vi "Forebrain.vi"() -> ()   [LabVIEW 2010]
doc: "This VI contrains the Forebrain within the Olin Robot Architecture. It must be run first to load the appropriate mission definition files. It contains a finite state machine built around a tabbed Operator interface that will guide an operator through the startup, run shutdown mission sequence. After running it, run the Midbrain and Hindbrain VIS."
panel:
  out "MDF_Original":T1(array[cluster])
  out "(xr,yr) A":cluster{"X":dbl, "Y":dbl}
  out "What?Midbrain":cluster{"T":dbl, "Range":dbl, "Bearing":dbl}[](array[cluster])
  out "How?Midbrain":cluster{"T":dbl, "Battery":dbl, "Temp":dbl}
  out "What?Forebrain":cluster{"T":dbl, "Range":dbl, "Bearing":dbl}[](array[cluster])
  out "How?Forebrain":cluster{"T":dbl, "Battery":dbl, "Temp":dbl}
  out "Where? Forebrain":T2
  out "WhereAmI? Clean":T2
  out "(xr,yr)":cluster{"X":dbl, "Y":dbl}
  out "How?ForebrainOut":cluster{"T":dbl, "Battery":dbl, "Temp":dbl}
  out "How?MidbrainMM":cluster{"T":dbl, "Battery":dbl, "Temp":dbl}
  out "WhereAmI?MidB":T2
  out "Where?Forebrain":T2
  out "WhatAroundMe?MidB":cluster{"T":dbl, "Range":dbl, "Bearing":dbl}[](array[cluster])
  in  "RunRobot":bool
  out "Robot Live":bool
  in  "E-Stop":bool
  in  "Tab":T3(tab)
  out "Boolean 3":bool
  in  "Test Tail":bool
  out "StartMissionMap":picture
  out "Boolean 2":bool
  out "Boolean":bool
  in  "Test Starboard Motor":bool
  in  "Test Port Motor":bool
  out "Motors Hot":bool
  out "BatteryState":dbl(slide) scale=16.0..24.0
  out "LIDARCheck":picture
  out "MissionTime S&S":dbl(knob) scale=0.0..10.0
  out "CollisionWarning":bool
  out "DebugLIDAR":picture
  in  "SubPosition":T4 {"xrobot" min=0.0 max=300.0; "yrobot" min=0.0 max=300.0; "heading" min=-7.0 max=7.0 step=0.01}
  in  "LIDARControl":T5
  out "LIDAR Data (r:pixel b:degrees)":cluster{"Range":dbl, "Bearing":dbl}[](array[cluster])
  in  "Stop DebugSENSE":bool
  out "MissionMap":picture
  out "MDF Out":T1(array[cluster])
  out "initialized MDF":T1(array[cluster])
  in  "MDFile":T6
  out "Way Point Index":i32
  out "InitialWaypoint":cluster{"X":i16, "Y":i16}
  in  "Pen Color":u32(colorbox)=15671808
  in  "Select Pen Attributes":T7={"Width"=1, "Style"=enum."Solid"}
  out "Draw??":bool
  out "ManualActCommand":dbl[](array[numeric])
  out "Hypo Out":cluster{"Motor1":i16, "Motor 2":i16}
  out "NeoActCom":dbl[](array[numeric])
  out "SteerAngle":dbl
  in  "Depth_Leg":dbl(slide) min=0.0 max=20.0 step=0.01
  out "MDF":T1(array[cluster])
  in  "Select Your Behavior":T8(ring)
  out "No. of Waypoints":i32
  in  "Exit Planning":bool
  out "MissionDefFile":picture
  in  "RobotSpeed_Leg":dbl(slide) min=0.0 max=4.0 step=0.01 scale=0.0..4.0
  out "BuildMDF":bool
  out "ActManual":bool
  in  "Steering":dbl(knob) min=-25.0 max=25.0 step=1.0 scale=15.0..-15.0
  out "MWhat?":bool
  out "Where? 2":bool
  out "How? 2":bool
  in  "ManualModeStop":bool
  out "ManualModeLIDAR":picture
  out "ManualMissionMap":picture
  out "CollisionLight":bool
  out "Temp Light":bool
  in  "LIDAR":bool
  in  "MAP":bool
  out "Battery":dbl(slide) scale=16.0..24.0
  in  "RobotSpeed":dbl(slide) scale=0.0..4.0
  out "MissionTime":dbl(knob) scale=0.0..10.0
  out "Roll":dbl(knob) scale=-90.0..90.0
  out "Pitch":dbl(slide) scale=-20.0..20.0
  out "Heading":cluster{dbl, dbl}(knob)={0.0, 34.390870865624734} scale=180.0..-180.0
  out "Speed":dbl(knob) scale=0.0..4.0
  in  "Reset":bool
  out "Ready":bool
  in  "Pause":bool
  in  "Rerun MDF":bool
  out "ATempLight":bool
  out "CollisionLight 2":bool
  out "Act":bool
  out "Hypo":bool
  out "Neo-C":bool
  out "How?":bool
  out "What?":bool
  out "A Pitch":dbl(slide) scale=-20.0..20.0
  out "A Roll":dbl(knob) scale=-90.0..90.0
  out "A Heading":cluster{dbl, dbl}(knob)={0.0, 34.390870865624734} scale=180.0..-180.0
  out "A Speed":dbl(knob) scale=0.0..4.0
  out "AutoBattery":dbl(slide) scale=16.0..24.0
  out "AutoModeLIDAR":picture
  out "AutoMissionMap":picture
  in  "RunAutoMode":bool
  out "MissionTimeAuto":dbl(knob) scale=0.0..10.0
  out "Where?":bool
  # "To run\nrobot,\nclick\narrow\nabove\n\nTo shut \noff \nrobot,\nclick \nbutton\nbelow."
  # "Operation Directions\n\n1)Click on Startup&\nShutdown tab.\n2) Click on Run \nArrow on menubar.\nRun Forebrain,\nMidbrain and Hindbrain.\n3) Select a mssion \nmap file when asked.\n4) Check robot is \nfully operational on\nStartup tab.\n5) Debug with debug\ntabs as required.\n6) Select ManualMode\ntab and test drive \nrobot.\n7) Select PlanMission\ntab and set up \nmission.\n8) Go to AutoMode\ntab and run mission."
  # "Turns off drive\nmotors"
  # "To operate:\n1) Run Forebrain.vi\n2) Run Midbrain.vi\n3) Run Hindbrain.vi"
  # "Use this tab\nto explore\nLIDAR\ndata and \noperation"
  # "Set \nX=130\nY=100\nto put\nrobot\nin center of\nMission\nMap"
  # "Set\nNumberOfBeams\nSensorRange\nNoise\nto\nview\nsimulated\nsensor\ndata"
  # "Directions:\n1) Select Robot Behavior for each mission leg.\n2) Select Robot Speed for leg.\n3) Select Robot Depth for leg.\n4) Click on robots current location for first waypoint.\n5) Hold down button and drag to next\nwaypoint. Click on next leg waypoint.\n6) Hold mouse button down and drag to \nnext waypoint. \n7) Click on next waypoint. Repeat for full mission.\n8) MDF will store up to 20 waypoints."
  # "MDF"
  # "Camera"
  # "AMM"
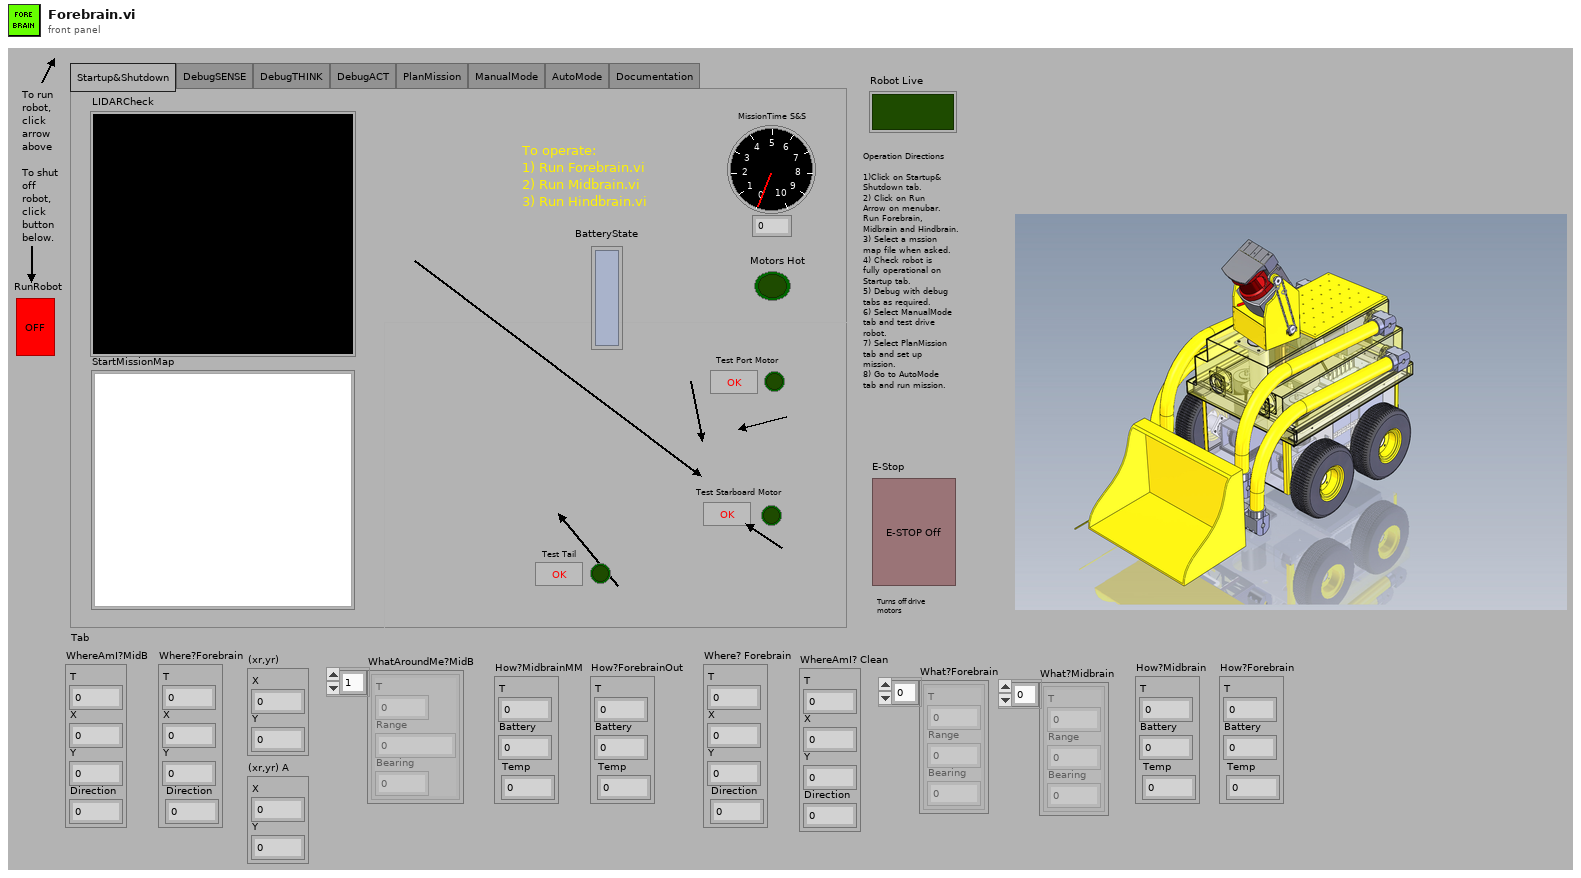
[diagram p1: front panel]
types:
  T1 = cluster{"Status":enum16{"Past", "Current", "Future"}, "x":dbl, "y":dbl, "z":dbl, "Vel":dbl, "Dwell Time":dbl, "Behavior":enum16{"OpenFieldTransit", "WallFollow", "LaneFollow", "ManualMode"}, "Expand1":dbl, "Expand2":dbl, "Expand3":dbl}[]
  T2 = cluster{"T":dbl, "X":dbl, "Y":dbl, "Direction":dbl}
  T3 = enum32{"Startup&Shutdown", "DebugSENSE", "DebugTHINK", "DebugACT", "PlanMission", "ManualMode", "AutoMode", "Documentation"}
  T4 = cluster{"xrobot":dbl, "yrobot":dbl, "heading":dbl}
  T5 = cluster{"NumberOfBeams":i32, "SensorRange":dbl, "Noise (0.1 to 1)":dbl}
  T6 = cluster{"Status":enum16{"Past", "Current", "Future"}, "x":dbl, "y":dbl, "z":dbl, "Vel":dbl, "Dwell Time":dbl, "Behavior":enum16{"OpenFieldTransit", "WallFollow", "LaneFollow", "ManualMode"}, "Expand1":dbl, "Expand2":dbl, "Expand3":dbl}
  T7 = cluster{"Width":u16, "Style":enum32{"Solid", "Dash", "Dot", "DashDot", "DashDotDot"}}
  T8 = enum16{"OpenFieldTransit", "WallFollow", "LaneFollow", "ManualMode"}
  T9 = cluster{"VelCom":dbl, "BehCom":enum16{"OpenFieldTransit", "WallFollow", "LaneFollow", "ManualMode"}}
  T10 = typedef "IMAQ Image.ctl" = refnum<image>
  T11 = typedef "imagedata.ctl" = cluster{"image type":i32, "image depth":i32, "image":u8[], "mask":u8[], "colors":u32[], "Rectangle":cluster{"left":i16, "top":i16, "right":i16, "bottom":i16}}
  T12 = typedef "LVMouseTypeDef.ctl" = cluster{"Mouse Position":cluster{"X":i32, "Y":i32}, "Mouse Modifiers":cluster{"Button Down":bool, "Shift Mod":bool, "Menu Mod":bool, "Option Mod":bool}}
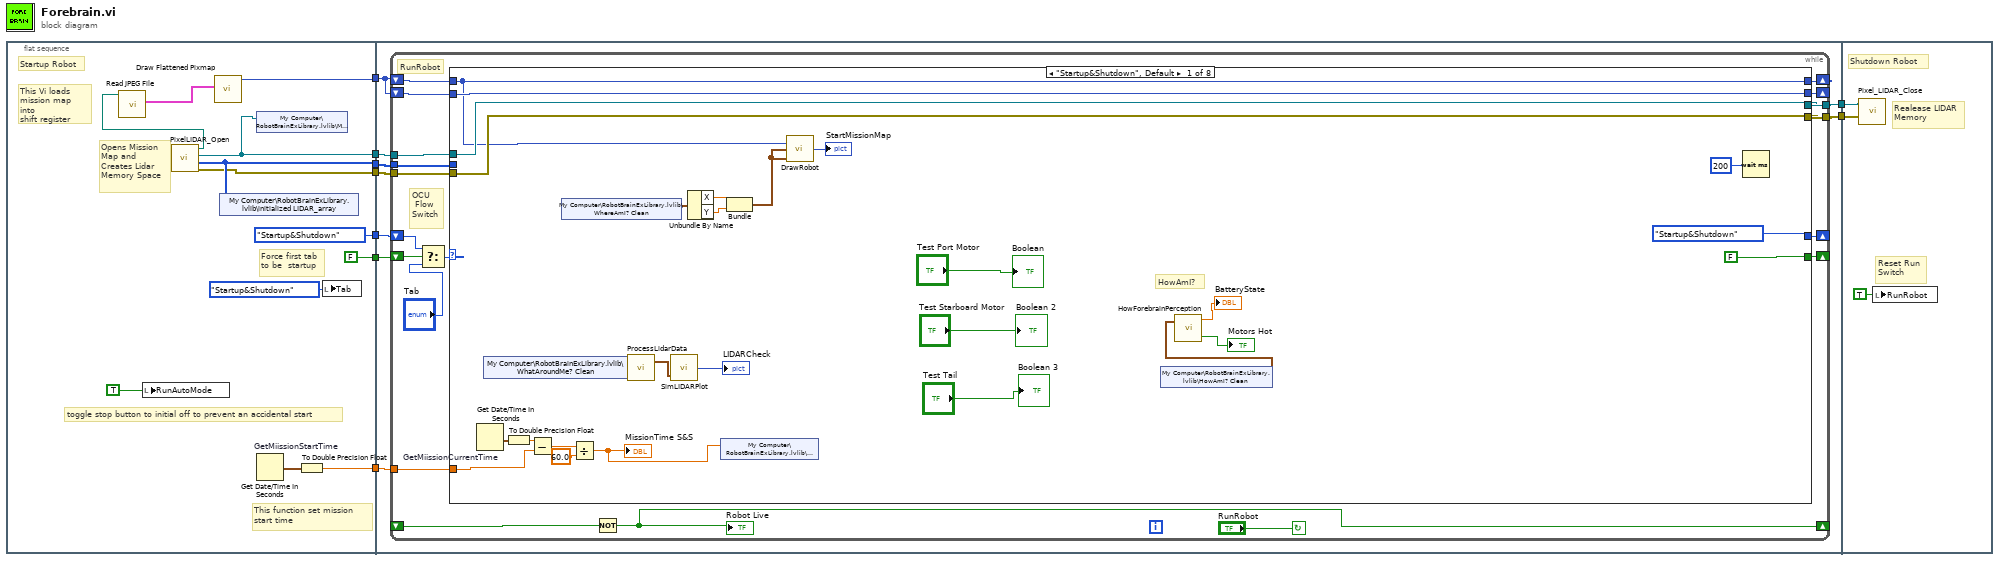
[diagram p0: block diagram]
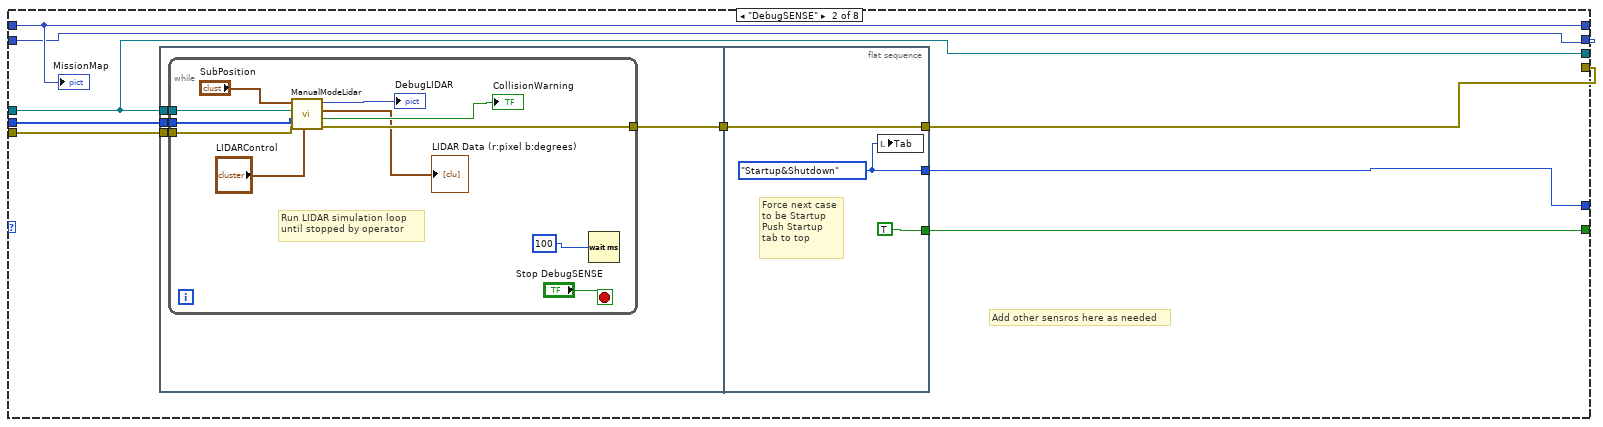
[diagram p2: hidden frame]
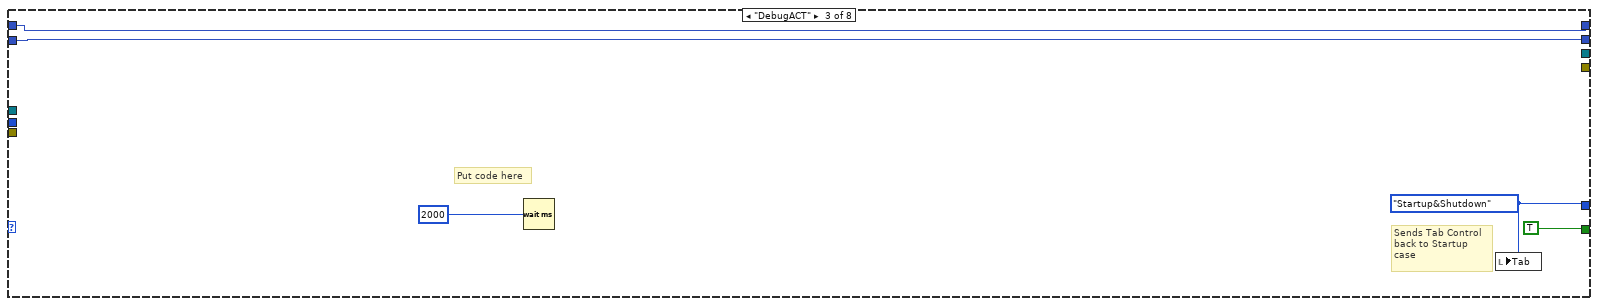
[diagram p3: hidden frame]
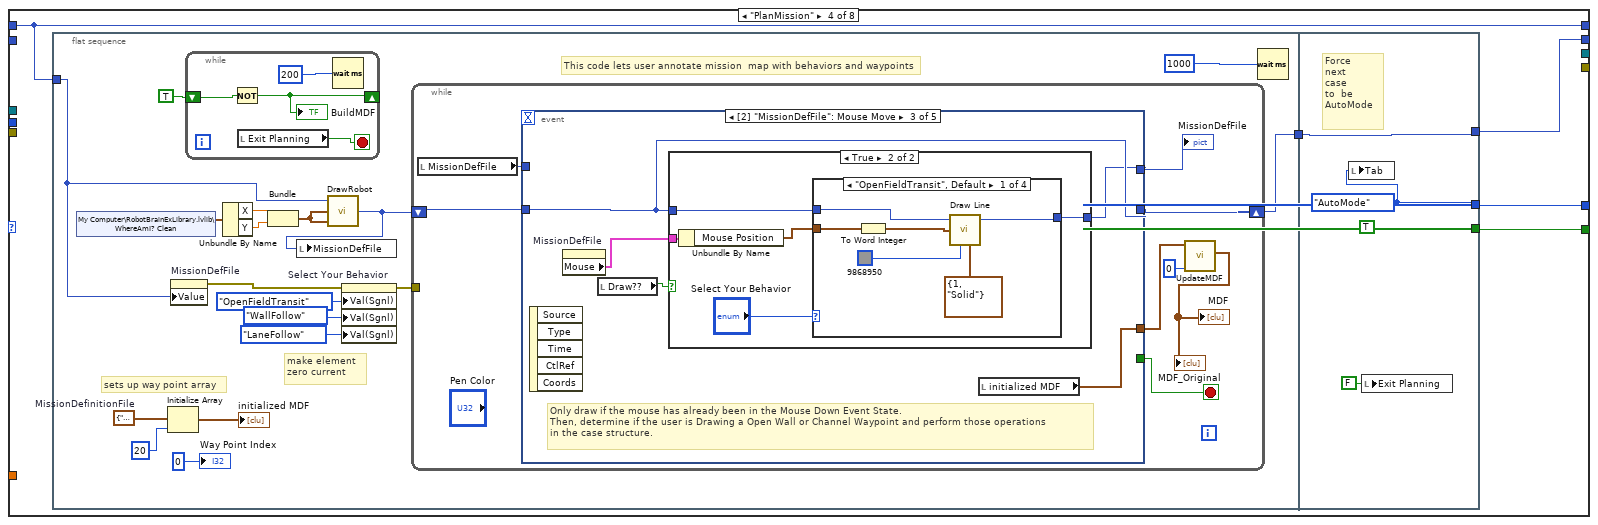
[diagram p4: hidden frame]
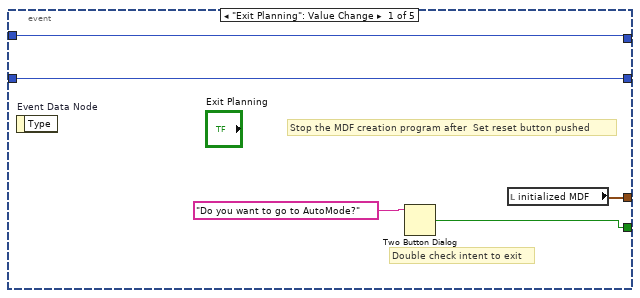
[diagram p5: hidden frame]
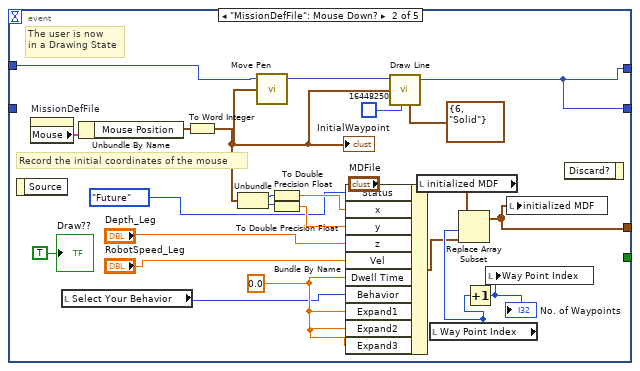
[diagram p6: hidden frame]
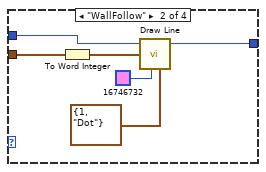
[diagram p8: hidden frame]
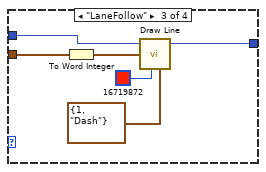
[diagram p9: hidden frame]
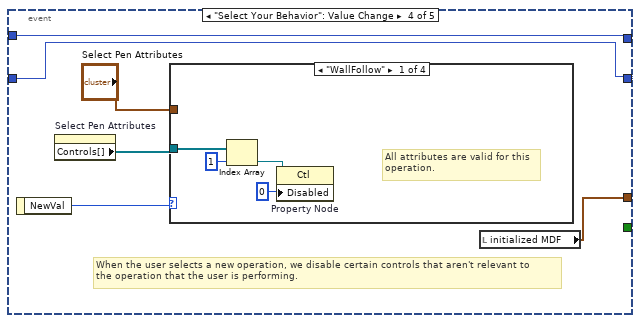
[diagram p11: hidden frame]
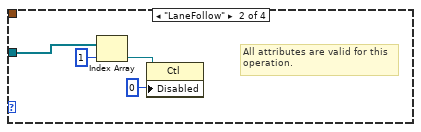
[diagram p12: hidden frame]
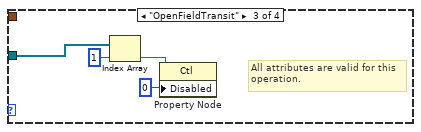
[diagram p13: hidden frame]
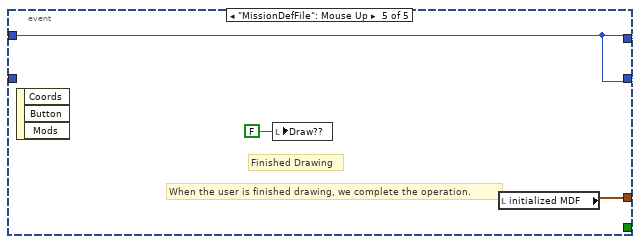
[diagram p15: hidden frame]
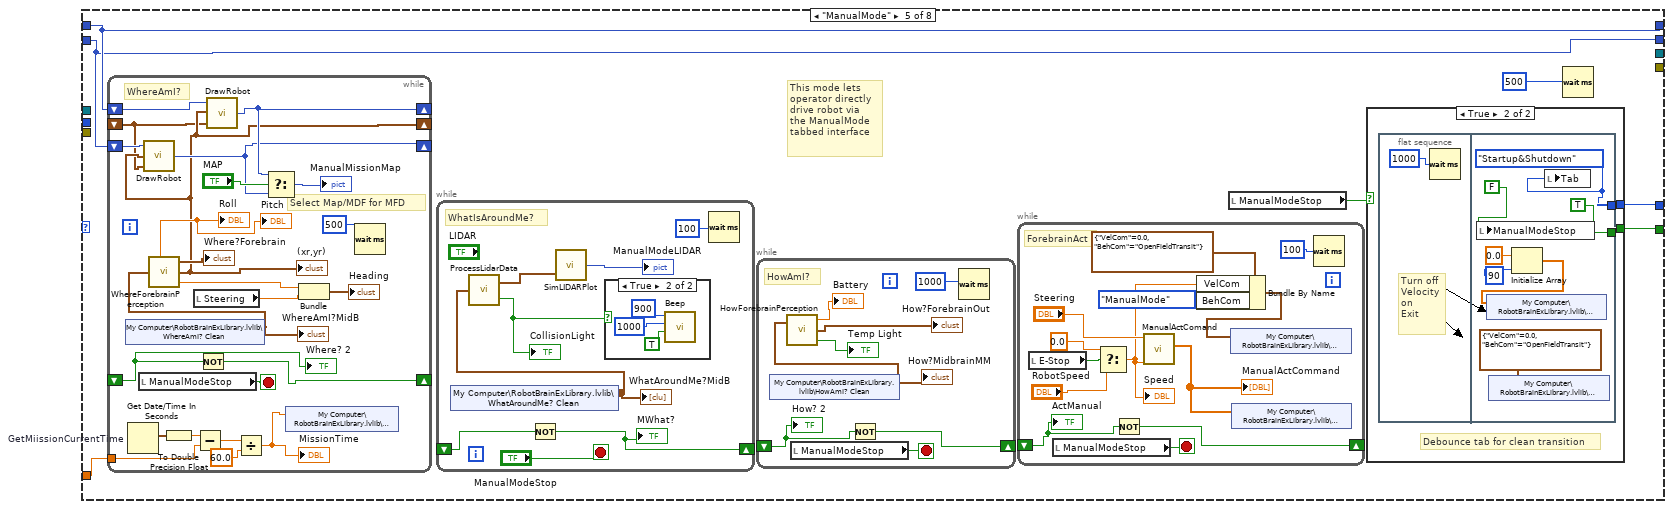
[diagram p16: hidden frame]
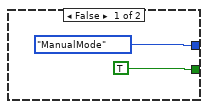
[diagram p18: hidden frame]
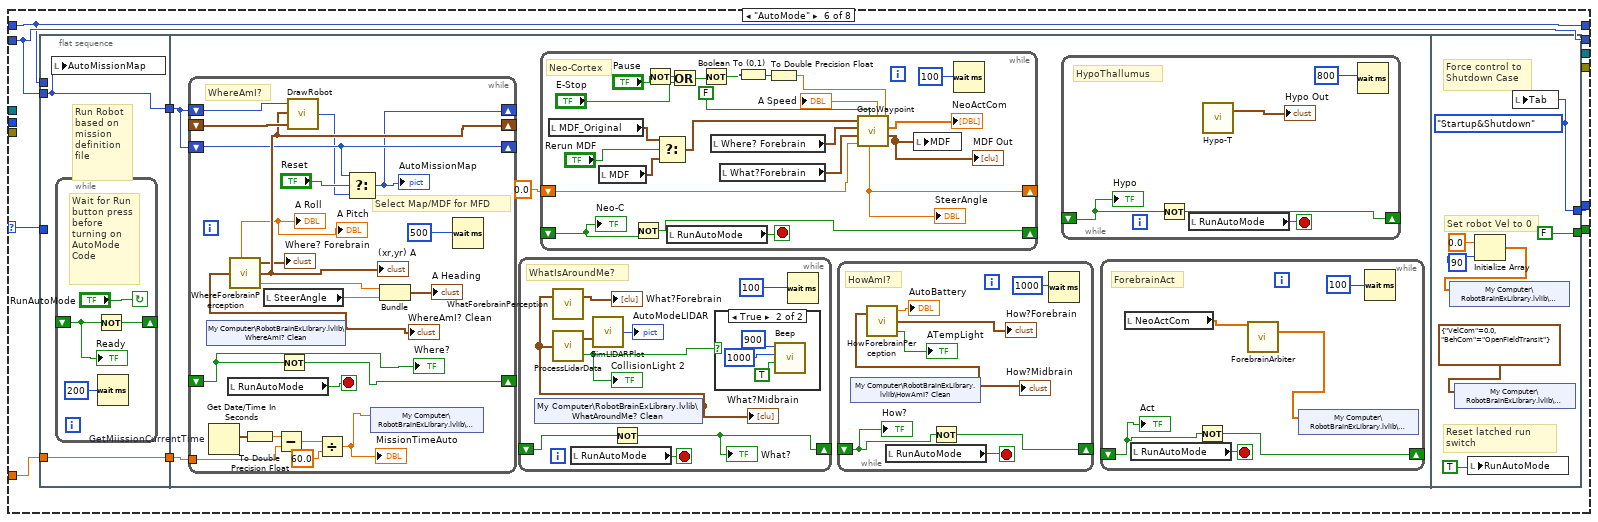
[diagram p19: hidden frame]
diagram:
  n1 = flat-sequence {
    tunnel: [w20] -> w9
    tunnel: [w18] -> w8
    tunnel: [w14] -> w7
    tunnel: [w16] -> w6
    tunnel: [w15] -> w5
    tunnel: [FALSE ("RunAutoMode")] -> w2
    tunnel: [T3."Startup&Shutdown" ("Tab")] -> w1
    tunnel: w9 -> [w30]
    tunnel: w8 -> [w29]
    tunnel: w7 -> [w28]
    tunnel: w6 -> [w27]
    tunnel: w5 -> [w26]
    tunnel: [w25] -> w4
    tunnel: [w24] -> w3
    tunnel: w2 -> [w23]
    tunnel: w1 -> [w22]
    tunnel: w4 -> [w415]
    tunnel: w3 -> [w414]
    frame #0 {
      # "Force first tab\nto be  startup"
      # "toggle stop button to initial off to prevent an accidental start"
      # "Opens Mission\nMap and\nCreates Lidar\nMemory Space"
      # "This function set mission \nstart time"
      # "This Vi loads\nmission map into \nshift register"
      # "Startup Robot"
      n2 = local write "RunAutoMode"(TRUE ("RunAutoMode")) -> ()
      n3 = call "PixelLIDAR_Open.vi"() -> ("error out"=w15:errorcluster, "initialized LIDAR\narray"=w16:i32[], "MDF Image"=w14:T10, "MissionMap"=w17:path)  [unwired: 2 in]
      n4 = call <vilib>:"Read JPEG File.vi"("path to JPEG file"=w17) -> ("image data"=w19:T11)  [unwired: 8 in, 2 out]
      n5 = call <vilib>:"Draw Flattened Pixmap.vi"("image data"=w19) -> ("new picture"=w18:picture)  [unwired: 8 in]
      n6 = shared-variable "My Computer\\RobotBrainExLibrary.lvlib\\initialized LIDAR_array"(w16) -> ()  [unwired: 1 in, 1 out]
      n7 = shared-variable "My Computer\\RobotBrainExLibrary.lvlib\\MDF Image"(w14) -> ()  [unwired: 1 in, 1 out]
      n8 = Get Date/Time In Seconds "GetMiissionStartTime"() -> (seconds since 1Jan1904=w21:timestamp)
      n9 = To Double Precision Float(number=w21) -> (double precision float=w20:dbl)
      n10 = local write "Tab"(T3."Startup&Shutdown" ("Tab")) -> ()
    }
    frame #1 {
      n11 = while {
        shift-right: [w31] -> _
        shift-left: _ -> [w48]
        shift-right: [w47] -> _
        shift-left: w22 -> [w46]
        shift-right: [w43] -> _
        shift-left: w23 -> [w42]
        tunnel: w30 -> [w41]
        shift-right: [w39] -> _
        shift-left: w29 -> [w40]
        shift-right: [w37] -> _
        shift-left: w29 -> [w38]
        tunnel: w28 -> [w36]
        tunnel: w27 -> [w35]
        tunnel: w26 -> [w34]
        tunnel: [w33] -> w25
        tunnel: [w32] -> w24
        stop <- "RunRobot" continue-if-true
        # "RunRobot"
        # "OCU\n Flow\nSwitch"
        n12 = Select(t=w46, s=w42, f="Tab") -> (s? t:f=w44:T3)
        n13 = case shown="\"Startup&Shutdown\", Default" w44 {
          selector: w44 -> [_ _ _ _ _ w309 _ _]
          tunnel: [T3."Startup&Shutdown" ("Tab") w80 w106 w113 w232 w310 T3."Startup&Shutdown" ("Tab") w412] -> w47
          tunnel: [FALSE ("s") w79 TRUE ("s") w112 w233 w308 FALSE ("s") TRUE ("s")] -> w43
          tunnel: w41 -> [w69 _ _ _ w230 w306 _ _]
          tunnel: w40 -> [w61 w82 w105 w109 w229 w303 w405 w410]
          tunnel: [w61 w82 w105 w109 w229 w303 w405 w410] -> w39
          tunnel: w38 -> [w68 w77 w104 _ w228 w305 w404 w409]
          tunnel: [w68 w77 w104 w110 w228 w305 w404 w409] -> w37
          tunnel: w36 -> [w67 w78 _ _ _ _ _ _]
          tunnel: w35 -> [_ w85 _ _ _ _ _ _]
          tunnel: w34 -> [w66 w84 _ _ _ _ _ _]
          tunnel: [w67 w78 _ _ _ _ _ _] -> w33
          tunnel: [w66 w83 _ _ _ _ _ _] -> w32
          frame "Startup&Shutdown", Default {
            # "HowAmI?"
            n14 = Get Date/Time In Seconds "GetMiissionCurrentTime"() -> (seconds since 1Jan1904=w73:timestamp)
            n15 = shared-variable "My Computer\\RobotBrainExLibrary.lvlib\\WhatAroundMe? Clean"() -> (w62:cluster{"T":dbl, "Range":dbl, "Bearing":dbl}[])  [unwired: 1 in, 1 out]
            n16 = To Double Precision Float(number=w73) -> (double precision float=w72:dbl)
            n17 = Subtract(x=w72, y=w69) -> (x-y=w71:dbl)
            n18 = shared-variable "My Computer\\RobotBrainExLibrary.lvlib\\WhereAmI? Clean"() -> (w54:T2)  [unwired: 1 in, 1 out]
            n19 = Divide(x=w71, y=60.0) -> (x/y=w65:dbl)
            "MissionTime S&S" <- w65
            n20 = call "ProcessLidarData.vi"("WhatAroundMe?MM"=w62) -> ("data array [mag, phase (deg)]"=w63:cluster{"magnitude":dbl, "phase":dbl}[])  [unwired: 1 out]
            n21 = call "SimLIDARPlot.vi"("data array [mag, phase (deg)]"=w63) -> ("SONAR"=→"LIDARCheck":picture)  [unwired: 1 in]
            n22 = Unbundle By Name(w54) -> ("X"=w53:dbl, "Y"=w52:dbl)
            n23 = shared-variable "My Computer\\RobotBrainExLibrary.lvlib\\MissionTime"(w65) -> ()  [unwired: 1 in, 1 out]
            n24 = Bundle("X"=w53, "Y"=w52) -> (w51:cluster{"X":dbl, "Y":dbl})  [unwired: 1 in]
            n25 = call "DrawRobot.vi"("(xr,yr) old"=w51, "(xr,yr) new"=w51, "2D Picture"=w61) -> ("new picture"=→"StartMissionMap":picture)
            n26 = shared-variable "My Computer\\RobotBrainExLibrary.lvlib\\HowAmI? Clean"() -> (w59:cluster{"T":dbl, "Battery":dbl, "Temp":dbl})  [unwired: 1 in, 1 out]
            n27 = call "HowForebrainPerception.vi"("How?MidbrainIn"=w59) -> ("TempWarning"=→"Motors Hot":bool, "BatteryGauge"=→"BatteryState":dbl)  [unwired: 1 in, 1 out]
            n28 = Wait (ms)(milliseconds to wait=u32 200) -> ()  [unwired: 1 out]
            "Boolean" <- "Test Port Motor"
            "Boolean 2" <- "Test Starboard Motor"
            "Boolean 3" <- "Test Tail"
          }
          frame "DebugSENSE" {
            # "Add other sensros here as needed"
            n29 = flat-sequence {
              tunnel: w85 -> [w89]
              tunnel: w84 -> [w88]
              tunnel: w78 -> [w87]
              tunnel: [w86] -> w81
              tunnel: [w103] -> w83
              tunnel: w81 -> [w103]
              tunnel: [w102] -> w80
              tunnel: [TRUE ("s")] -> w79
              frame #0 {
                n30 = while {
                  tunnel: w89 -> [w100]
                  tunnel: w88 -> [w99]
                  tunnel: w87 -> [w98]
                  tunnel: [w97] -> w86
                  stop <- "Stop DebugSENSE" stop-if-true
                  # "Run LIDAR simulation loop\nuntil stopped by operator"
                  n31 = call "ManualModeLidar.vi"("LIDARControl"="LIDARControl", "error in"=w99, "initialized \nsonar ray\narray"=w100, "MDF Image"=w98, "SubPosition"="SubPosition") -> ("error out"=w97:errorcluster, "Collision\nWarning"=→"CollisionWarning":bool, "LIDAR Data (r:pixel b:degrees)"=→"LIDAR Data (r:pixel b:degrees)":cluster{"Range":dbl, "Bearing":dbl}[], "LIDAR"=→"DebugLIDAR":picture)  [unwired: 1 in]
                  n32 = Wait (ms)(milliseconds to wait=u32 100) -> ()  [unwired: 1 out]
                }
              }
              frame #1 {
                w102 = T3."Startup&Shutdown" ("Tab")
                # "Force next case\nto be Startup\nPush Startup\ntab to top"
                n33 = local write "Tab"(w102) -> ()
              }
            }
            "MissionMap" <- w82
          }
          frame "DebugACT" {
            w106 = T3."Startup&Shutdown" ("Tab")
            # "Put code here"
            # "Sends Tab Control\nback to Startup\ncase"
            n34 = Wait (ms)(milliseconds to wait=u32 2000) -> ()  [unwired: 1 out]
            n35 = local write "Tab"(w106) -> ()
          }
          frame "PlanMission" {
            n36 = flat-sequence {
              tunnel: [w130] -> w111
              tunnel: w109 -> [w115]
              tunnel: [w226] -> w113
              tunnel: [TRUE ("s")] -> w112
              tunnel: w111 -> [w225]
              tunnel: [w225] -> w110
              frame #0 {
                w125 = T6 {"Status"=enum."Future", "x"=0.0, "y"=0.0, "z"=0.0, "Vel"=0.0, "Dwell Time"=0.0, "Behavior"=enum."OpenFieldTransit", "Expand1"=0.0, "Expand2"=0.0, "Expand3"=0.0}  # MissionDefinitionFile
                # "make element \nzero current"
                # "sets up way point array"
                # "This code lets user annotate mission  map with behaviors and waypoints"
                n37 = shared-variable "My Computer\\RobotBrainExLibrary.lvlib\\WhereAmI? Clean"() -> (w119:T2)  [unwired: 1 in, 1 out]
                n38 = Initialize Array ("Initialize WaypointArray")(w125, 20 ("dimension size")) -> (→"initialized MDF":T1)
                n39 = property on="MissionDefFile" class="Pict"("Value"=w115) -> (error out=w128:errorcluster)  [unwired: 2 in, 1 out]
                n40 = while {
                  shift-right: [w134] -> _
                  shift-left: TRUE -> [w135]
                  stop <- w133 stop-if-true
                  n41 = Not(x=w135) -> (.not. x?=w134:bool)
                  "BuildMDF" <- w134
                  n42 = local read "Exit Planning"() -> (w133:bool)
                  n43 = Wait (ms)(milliseconds to wait=u32 200) -> ()  [unwired: 1 out]
                }
                n44 = Unbundle By Name(w119) -> ("X"=w118:dbl, "Y"=w117:dbl)
                n45 = Bundle("X"=w118, "Y"=w117) -> (w116:cluster{"X":dbl, "Y":dbl})  [unwired: 1 in]
                n46 = call "DrawRobot.vi"("(xr,yr) old"=w116, "(xr,yr) new"=w116, "2D Picture"=w115) -> ("new picture"=w114:picture)
                n47 = local write "MissionDefFile"(w114) -> ()
                n48 = property on="Select Your Behavior" class="Enum (strict)"(error in=w128, "Val(Sgnl)"=T8."OpenFieldTransit" ("Select Your Behavior"), "Val(Sgnl)"=T8."WallFollow" ("Value (Signaling)"), "Val(Sgnl)"=T8."LaneFollow" ("Select Your Behavior")) -> (error out=w129:errorcluster)  [unwired: 1 in, 1 out]
                n49 = while {
                  shift-right: [w142] -> w130
                  shift-left: w114 -> [w143]
                  tunnel: w129 -> [_]
                  stop <- w141 stop-if-true
                  n50 = local read "MissionDefFile"() -> (w140:picture)
                  n51 = event shown="[2] \"MissionDefFile\": Mouse Move" {
                    selector: _ -> [_ _ _ _ _]
                    dyn-events: _ -> [_ _ _ _ _]
                    timeout: _ -> [_ _ _ _ _]
                    tunnel: [w146 w149 w174 w203 w221] -> w142
                    tunnel: w143 -> [w146 _ w174 w203 _]
                    tunnel: [w147 _ _ _ _] -> w141
                    tunnel: [w145 w169 w175 w205 w222] -> w138
                    tunnel: w140 -> [w144 w150 _ w204 w221]
                    tunnel: [w144 w149 w173 w204 w221] -> w139
                    event "Exit Planning": Value Change {
                      # "Double check intent to exit"
                      # "Stop the MDF creation program after  Set reset button pushed"
                      n52 = event-data "Event Data Node"() -> ()  [unwired: 1 in, 1 out]
                      n53 = Two Button Dialog(message="Do you want to go to AutoMode?") -> (T button?=w147:bool)  [unwired: 2 in]
                      n54 = local read "initialized MDF"() -> (w145:T1)
                    }
                    event "MissionDefFile": Mouse Down? {
                      w160 = 0.0 ("Dwell Time")
                      # "Record the initial coordinates of the mouse"
                      # "The user is now\nin a Drawing State"
                      n55 = event-data() -> ()  [unwired: 1 in, 1 out]
                      n56 = property on="MissionDefFile" class="Pict"() -> ("Mouse"=w172:T12)  [unwired: 2 in, 2 out]
                      n57 = local read "Select Your Behavior"() -> (w159:T8)
                      n58 = Unbundle By Name(w172) -> ("Mouse Position"=w170:cluster{"X":i32, "Y":i32})
                      n59 = To Word Integer(number=w170) -> (16bit integer=w153:cluster{"X":i16, "Y":i16})
                      "InitialWaypoint" <- w153
                      n60 = Unbundle(w153) -> ("X"=w164:i16, "Y"=w163:i16)
                      n61 = call <vilib>:"Move Pen.vi"("new position"=w153, "picture"=w150) -> ("new picture"=w154:picture)  [unwired: 3 in]
                      n62 = To Double Precision Float(number=w164) -> (double precision float=w162:dbl)
                      n63 = To Double Precision Float(number=w163) -> (double precision float=w161:dbl)
                      n64 = Bundle By Name(cluster="MDFile", "Status"=enum16{"Past", "Current", "Future"}."Future", "x"=w162, "y"=w161, "z"="Depth_Leg", "Vel"="RobotSpeed_Leg", "Dwell Time"=w160, "Behavior"=w159, "Expand1"=w160, "Expand2"=w160, "Expand3"=w160) -> (w165:T6)
                      n65 = call <vilib>:"Draw Line.vi"("picture"=w154, "end point"=w153, "color(black)"=u32 16448250, "pen"=T7 {"Width"=6, "Style"=enum."Solid"}) -> ("new picture"=w149:picture)  [unwired: 5 in]
                      n66 = local read "initialized MDF"() -> (w167:T1)
                      n67 = local read "Way Point Index"() -> (w168:i32)
                      n68 = Replace Array Subset(array=w167, new element=w165, index=w168) -> (w169:T1)
                      n69 = Increment(x=w168) -> (x+1=w171:i32)
                      "No. of Waypoints" <- w171
                      n70 = local write "Way Point Index"(w171) -> ()
                      n71 = local write "initialized MDF"(w169) -> ()
                      n72 = event-data() -> ()  [unwired: 2 in, 1 out]
                      "Draw??" <- TRUE ("Draw??")
                    }
                    event "MissionDefFile": Mouse Move {
                      # "Only draw if the mouse has already been in the Mouse Down Event State.\nThen, determine if the user is Drawing a Open Wall or Channel Waypoint and perform those operations\nin the case structure."
                      n73 = event-data() -> ()  [unwired: 1 in, 5 out]
                      n74 = property on="MissionDefFile" class="Pict"() -> ("Mouse"=w177:T12)  [unwired: 2 in, 2 out]
                      n75 = local read "Draw??"() -> (w176:bool)
                      n76 = case shown="True" w176 {
                        tunnel: w177 -> [_ w183]
                        tunnel: w174 -> [w178 w180]
                        tunnel: [w178 w179] -> w173
                        frame False {
                        }
                        frame True {
                          n77 = Unbundle By Name(w183) -> ("Mouse Position"=w181:cluster{"X":i32, "Y":i32})
                          n78 = case shown="\"OpenFieldTransit\", Default" "Select Your Behavior" {
                            tunnel: w181 -> [w187 w194 w200 _]
                            tunnel: [w188 w195 w201 w202] -> w179
                            tunnel: w180 -> [w189 w193 w197 w202]
                            frame "OpenFieldTransit", Default {
                              n79 = To Word Integer(number=w187) -> (16bit integer=w186:cluster{"X":i16, "Y":i16})
                              n80 = call <vilib>:"Draw Line.vi"("picture"=w189, "end point"=w186, "color(black)"=u32 9868950, "pen"=T7 {"Width"=1, "Style"=enum."Solid"}) -> ("new picture"=w188:picture)  [unwired: 5 in]
                            }
                            frame "WallFollow" {
                              n81 = To Word Integer(number=w194) -> (16bit integer=w190:cluster{"X":i16, "Y":i16})
                              n82 = call <vilib>:"Draw Line.vi"("picture"=w193, "end point"=w190, "color(black)"=u32 16746732, "pen"=T7 {"Width"=1, "Style"=enum."Dot"}) -> ("new picture"=w195:picture)  [unwired: 5 in]
                            }
                            frame "LaneFollow" {
                              n83 = To Word Integer(number=w200) -> (16bit integer=w196:cluster{"X":i16, "Y":i16})
                              n84 = call <vilib>:"Draw Line.vi"("picture"=w197, "end point"=w196, "color(black)"=u32 16719872, "pen"=T7 {"Width"=1, "Style"=enum."Dash"}) -> ("new picture"=w201:picture)  [unwired: 5 in]
                            }
                            frame "ManualMode" {
                            }
                          }
                        }
                      }
                      n85 = local read "initialized MDF"() -> (w175:T1)
                    }
                    event "Select Your Behavior": Value Change {
                      # "When the user selects a new operation, we disable certain controls that aren't relevant to\nthe operation that the user is performing."
                      n86 = event-data() -> ("NewVal"=w208:T8)  [unwired: 1 in]
                      n87 = property on="Select Pen Attributes" class="Clust (strict)"() -> ("Controls[]"=w207:refnum<vi>[])  [unwired: 2 in, 2 out]
                      n88 = case shown="\"WallFollow\"" w208 {
                        tunnel: w207 -> [w212 w213 w217 _]
                        tunnel: "Select Pen Attributes" -> [_ _ _ _]
                        frame "WallFollow" {
                          # "All attributes are valid for this\noperation."
                          n89 = Index Array "Index Array"(array=w212, index=1) -> (element=w210:refnum<vi>)
                          n90 = property on="Property Node" class="Ctl"(reference=w210, "Disabled"=u8 0) -> ()  [unwired: 1 in, 2 out]
                        }
                        frame "LaneFollow" {
                          # "All attributes are valid for this\noperation."
                          n91 = Index Array(array=w213, index=1) -> (element=w215:refnum<vi>)
                          n92 = property class="Ctl"(reference=w215, "Disabled"=u8 0) -> ()  [unwired: 1 in, 2 out]
                        }
                        frame "OpenFieldTransit" {
                          # "All attributes are valid for this\noperation."
                          n93 = Index Array "Index Array"(array=w217, index=1) -> (element=w219:refnum<vi>)
                          n94 = property on="Property Node" class="Ctl"(reference=w219, "Disabled"=u8 0) -> ()  [unwired: 1 in, 2 out]
                        }
                        frame "ManualMode" {
                        }
                      }
                      n95 = local read "initialized MDF"() -> (w205:T1)
                    }
                    event "MissionDefFile": Mouse Up {
                      # "When the user is finished drawing, we complete the operation."
                      # "Finished Drawing"
                      n96 = event-data() -> ()  [unwired: 1 in, 3 out]
                      n97 = local write "Draw??"(FALSE ("Draw??")) -> ()
                      n98 = local read "initialized MDF"() -> (w222:T1)
                    }
                  }
                  "MissionDefFile" <- w139
                  n99 = call "UpdateMDF.vi"("Index"=0, "MDF_In"=w138) -> ("MDF_Out"=→"MDF" →"MDF_Original":T1)  [unwired: 9 in]
                }
                n100 = Wait (ms)(milliseconds to wait=u32 1000) -> ()  [unwired: 1 out]
                "Way Point Index" <- 0 ("Boundary Point Index")
              }
              frame #1 {
                w226 = T3."AutoMode" ("Tab")
                # "Force \nnext \ncase\nto  be\nAutoMode"
                n101 = local write "Tab"(w226) -> ()
                n102 = local write "Exit Planning"(FALSE ("Exit Planning")) -> ()
              }
            }
          }
          frame "ManualMode" {
            # "This mode lets \noperator directly\ndrive robot via\nthe ManualMode\ntabbed interface"
            n103 = while {
              shift-right: [w257] -> _
              shift-left: _ -> [w256]
              tunnel: w230 -> [w249]
              shift-right: [w239] -> _
              shift-left: w229 -> [w242]
              shift-right: [w236] -> _
              shift-left: _ -> [w235]
              shift-right: [w237] -> _
              shift-left: w228 -> [w238]
              stop <- w255 stop-if-true
              # "Select Map/MDF for MFD"
              # "WhereAmI?"
              n104 = shared-variable "My Computer\\RobotBrainExLibrary.lvlib\\WhereAmI? Clean"() -> (w248:T2)  [unwired: 1 in, 1 out]
              "WhereAmI?MidB" <- w248
              n105 = Get Date/Time In Seconds "GetMiissionCurrentTime"() -> (seconds since 1Jan1904=w250:timestamp)
              n106 = local read "ManualModeStop"() -> (w255:bool)
              n107 = call "WhereForebrainPerception.vi"("Where? Midbrain"=w248) -> ("SimPitchRoll"=→"Roll" →"Pitch":dbl, "Where? Forebrain"=→"Where?Forebrain":T2, "(xr,yr)"=w236:cluster{"X":dbl, "Y":dbl}, "Direction"=w246:dbl)  [unwired: 3 in]
              "(xr,yr)" <- w236
              n108 = call "DrawRobot.vi"("(xr,yr) old"=w235, "(xr,yr) new"=w236, "2D Picture"=w238) -> ("new picture"=w237:picture)
              n109 = To Double Precision Float(number=w250) -> (double precision float=w251:dbl)
              n110 = local read "Steering"() -> (w244:dbl)
              n111 = Subtract(x=w251, y=w249) -> (x-y=w252:dbl)
              n112 = Not(x=w256) -> (.not. x?=w257:bool)
              n113 = call "DrawRobot.vi"("(xr,yr) old"=w235, "(xr,yr) new"=w236, "2D Picture"=w242) -> ("new picture"=w239:picture)
              n114 = Divide(x=w252, y=60.0) -> (x/y=w254:dbl)
              "MissionTime" <- w254
              n115 = Select(t=w239, s="MAP", f=w237) -> (s? t:f=→"ManualMissionMap":picture)
              n116 = shared-variable "My Computer\\RobotBrainExLibrary.lvlib\\MissionTime"(w254) -> ()  [unwired: 1 in, 1 out]
              n117 = Bundle("Direction"=w246, "Steering"=w244) -> (→"Heading":cluster{"Direction":dbl, "Steering":dbl})  [unwired: 1 in]
              n118 = Wait (ms)(milliseconds to wait=u32 500) -> ()  [unwired: 1 out]
              "Where? 2" <- w256
            }
            n119 = while {
              shift-right: [w264] -> _
              shift-left: _ -> [w265]
              stop <- "ManualModeStop" stop-if-true
              # "WhatIsAroundMe?"
              n120 = shared-variable "My Computer\\RobotBrainExLibrary.lvlib\\WhatAroundMe? Clean"() -> (w260:cluster{"T":dbl, "Range":dbl, "Bearing":dbl}[])  [unwired: 1 in, 1 out]
              "WhatAroundMe?MidB" <- w260
              n121 = call "ProcessLidarData.vi"("WhatAroundMe?MM"=w260) -> ("Collision"=w259:bool, "data array [mag, phase (deg)]"=w261:cluster{"magnitude":dbl, "phase":dbl}[])
              "CollisionLight" <- w259
              n122 = Not(x=w265) -> (.not. x?=w264:bool)
              "MWhat?" <- w264
              n123 = call "SimLIDARPlot.vi"("data array [mag, phase (deg)]"=w261) -> ("SONAR"=→"ManualModeLIDAR":picture)  [unwired: 1 in]
              n124 = case shown="True" w259 {
                frame False {
                  # "No \nBeep"
                }
                frame True {
                  n125 = call <vilib>:"Beep.vi"("use system alert? (T)"=TRUE, "duration (msec)"=u32 1000, "frequency (Hz)"=u32 900) -> ()  [unwired: 9 in]
                }
              }
              n126 = Wait (ms)(milliseconds to wait=u32 100) -> ()  [unwired: 1 out]
            }
            n127 = while {
              shift-right: [w289] -> _
              shift-left: _ -> [w288]
              stop <- w283 stop-if-true
              # "HowAmI?"
              n128 = shared-variable "My Computer\\RobotBrainExLibrary.lvlib\\HowAmI? Clean"() -> (w287:cluster{"T":dbl, "Battery":dbl, "Temp":dbl})  [unwired: 1 in, 1 out]
              "How?MidbrainMM" <- w287
              n129 = call "HowForebrainPerception.vi"("How?MidbrainIn"=w287) -> ("TempWarning"=→"Temp Light":bool, "How?ForebrainOut"=→"How?ForebrainOut":cluster{"T":dbl, "Battery":dbl, "Temp":dbl}, "BatteryGauge"=→"Battery":dbl)  [unwired: 1 in]
              n130 = local read "ManualModeStop"() -> (w283:bool)
              n131 = Not(x=w288) -> (.not. x?=w289:bool)
              n132 = Wait (ms)(milliseconds to wait=u32 1000) -> ()  [unwired: 1 out]
              "How? 2" <- w288
            }
            n133 = while {
              shift-right: [w281] -> _
              shift-left: _ -> [w280]
              stop <- w278 stop-if-true
              # "ForebrainAct"
              n134 = local read "E-Stop"() -> (w271:bool)
              n135 = local read "ManualModeStop"() -> (w278:bool)
              n136 = Select(t=0.0, s=w271, f="RobotSpeed") -> (s? t:f=w273:dbl)
              "Speed" <- w273
              n137 = Not(x=w280) -> (.not. x?=w281:bool)
              n138 = call "ManualActComand.vi"("Speed"=w273, "SteeringAngle"="Steering") -> ("ManualActCommand"=w279:dbl[])  [unwired: 9 in]
              "ManualActCommand" <- w279
              n139 = Bundle By Name(cluster=T9 {"VelCom"=0.0, "BehCom"=enum."OpenFieldTransit"} ("ForebrainCom"), "VelCom"=w273, "BehCom"=T8."ManualMode") -> (w276:T9)
              n140 = shared-variable "My Computer\\RobotBrainExLibrary.lvlib\\ForebrainCom"(w276) -> ()  [unwired: 1 in, 1 out]
              n141 = shared-variable "My Computer\\RobotBrainExLibrary.lvlib\\ActCommand"(w279) -> ()  [unwired: 1 in, 1 out]
              n142 = Wait (ms)(milliseconds to wait=u32 100) -> ()  [unwired: 1 out]
              "ActManual" <- w280
            }
            n143 = local read "ManualModeStop"() -> (w231:bool)
            n144 = case shown="True" w231 {
              tunnel: [TRUE ("s") w293] -> w233
              tunnel: [T3."ManualMode" ("Tab") w294] -> w232
              frame False {
              }
              frame True {
                # "Debounce tab for clean transition"
                n145 = flat-sequence {
                  tunnel: [w301] -> w294
                  tunnel: [TRUE ("s")] -> w293
                  frame #0 {
                    # "Turn off\nVelocity\non \nExit"
                    n146 = Wait (ms)(milliseconds to wait=u32 1000) -> ()  [unwired: 1 out]
                  }
                  frame #1 {
                    w301 = T3."Startup&Shutdown" ("Tab")
                    n147 = local write "ManualModeStop"(FALSE ("ManualModeStop")) -> ()
                    n148 = shared-variable "My Computer\\RobotBrainExLibrary.lvlib\\ForebrainCom"(T9 {"VelCom"=0.0, "BehCom"=enum."OpenFieldTransit"} ("ForebrainCom")) -> ()  [unwired: 1 in, 1 out]
                    n149 = Initialize Array(0.0 ("element"), 90 ("dimension size")) -> (w299:dbl[])
                    n150 = shared-variable "My Computer\\RobotBrainExLibrary.lvlib\\ActCommand"(w299) -> ()  [unwired: 1 in, 1 out]
                    n151 = local write "Tab"(w301) -> ()
                  }
                }
              }
            }
            n152 = Wait (ms)(milliseconds to wait=u32 500) -> ()  [unwired: 1 out]
          }
          frame "AutoMode" {
            n153 = flat-sequence {
              tunnel: w309 -> [_]
              tunnel: [w312] -> w307
              tunnel: w306 -> [w312]
              tunnel: w305 -> [w311]
              tunnel: [w311] -> w304
              tunnel: w303 -> [_]
              tunnel: w307 -> [w319]
              tunnel: w304 -> [w317]
              tunnel: [w402] -> w310
              tunnel: [FALSE ("s")] -> w308
              frame #0 {
                # "Run Robot\nbased on\nmission\ndefinition\nfile"
                n154 = local write "AutoMissionMap"(w311) -> ()
                n155 = while {
                  shift-right: [w315] -> _
                  shift-left: _ -> [w314]
                  stop <- "RunAutoMode" continue-if-true
                  # "Wait for Run\nbutton press\nbefore\nturning on\nAutoMode\nCode"
                  n156 = Not(x=w314) -> (.not. x?=w315:bool)
                  n157 = Wait (ms)(milliseconds to wait=u32 200) -> ()  [unwired: 1 out]
                  "Ready" <- w314
                }
              }
              frame #1 {
                n158 = while {
                  shift-right: [w372] -> _
                  shift-left: _ -> [w359]
                  tunnel: w319 -> [w367]
                  shift-right: [w351] -> _
                  shift-left: w317 -> [w354]
                  shift-right: [w364] -> _
                  shift-left: _ -> [w365]
                  shift-right: [w353] -> _
                  shift-left: w317 -> [w353]
                  stop <- w358 stop-if-true
                  # "Select Map/MDF for MFD"
                  # "WhereAmI?"
                  n159 = shared-variable "My Computer\\RobotBrainExLibrary.lvlib\\WhereAmI? Clean"() -> (w361:T2)  [unwired: 1 in, 1 out]
                  "WhereAmI? Clean" <- w361
                  n160 = Get Date/Time In Seconds "GetMiissionCurrentTime"() -> (seconds since 1Jan1904=w368:timestamp)
                  n161 = local read "RunAutoMode"() -> (w358:bool)
                  n162 = call "WhereForebrainPerception.vi"("Where? Midbrain"=w361) -> ("SimPitchRoll"=→"A Roll" →"A Pitch":dbl, "Where? Forebrain"=→"Where? Forebrain":T2, "(xr,yr)"=w364:cluster{"X":dbl, "Y":dbl}, "Direction"=w366:dbl)  [unwired: 3 in]
                  "(xr,yr) A" <- w364
                  n163 = To Double Precision Float(number=w368) -> (double precision float=w369:dbl)
                  n164 = local read "SteerAngle"() -> (w355:dbl)
                  n165 = Subtract(x=w369, y=w367) -> (x-y=w370:dbl)
                  n166 = Not(x=w359) -> (.not. x?=w372:bool)
                  n167 = call "DrawRobot.vi"("(xr,yr) old"=w365, "(xr,yr) new"=w364, "2D Picture"=w354) -> ("new picture"=w352:picture)
                  n168 = Divide(x=w370, y=60.0) -> (x/y=w360:dbl)
                  "MissionTimeAuto" <- w360
                  n169 = Select(t=w353, s="Reset", f=w352) -> (s? t:f=w351:picture)
                  "AutoMissionMap" <- w351
                  n170 = shared-variable "My Computer\\RobotBrainExLibrary.lvlib\\MissionTime"(w360) -> ()  [unwired: 1 in, 1 out]
                  n171 = Bundle("Direction"=w366, "SteerAngle"=w355) -> (→"A Heading":cluster{"Direction":dbl, "SteerAngle":dbl})  [unwired: 1 in]
                  n172 = Wait (ms)(milliseconds to wait=u32 500) -> ()  [unwired: 1 out]
                  "Where?" <- w359
                }
                n173 = while {
                  shift-right: [w344] -> _
                  shift-left: _ -> [w346]
                  stop <- w343 stop-if-true
                  # "WhatIsAroundMe?"
                  n174 = shared-variable "My Computer\\RobotBrainExLibrary.lvlib\\WhatAroundMe? Clean"() -> (w341:cluster{"T":dbl, "Range":dbl, "Bearing":dbl}[])  [unwired: 1 in, 1 out]
                  "What?Midbrain" <- w341
                  n175 = call "WhatForebrainPerception.vi"("What?Midbrain"=w341) -> ("What?Midbrain 2"=→"What?Forebrain":cluster{"T":dbl, "Range":dbl, "Bearing":dbl}[])  [unwired: 2 in]
                  n176 = call "ProcessLidarData.vi"("WhatAroundMe?MM"=w341) -> ("Collision"=w339:bool, "data array [mag, phase (deg)]"=w345:cluster{"magnitude":dbl, "phase":dbl}[])
                  "CollisionLight 2" <- w339
                  n177 = local read "RunAutoMode"() -> (w343:bool)
                  n178 = call "SimLIDARPlot.vi"("data array [mag, phase (deg)]"=w345) -> ("SONAR"=→"AutoModeLIDAR":picture)  [unwired: 1 in]
                  n179 = Not(x=w346) -> (.not. x?=w344:bool)
                  "What?" <- w344
                  n180 = case shown="True" w339 {
                    frame False {
                      # "No \nBeep"
                    }
                    frame True {
                      n181 = call <vilib>:"Beep.vi"("use system alert? (T)"=TRUE, "duration (msec)"=u32 1000, "frequency (Hz)"=u32 900) -> ()  [unwired: 9 in]
                    }
                  }
                  n182 = Wait (ms)(milliseconds to wait=u32 100) -> ()  [unwired: 1 out]
                }
                n183 = while {
                  shift-right: [w394] -> _
                  shift-left: _ -> [w393]
                  shift-right: [w386] -> _
                  shift-left: 0.0 ("SteerAngle") -> [w385]
                  stop <- w396 stop-if-true
                  # "Neo-Cortex"
                  n184 = local read "MDF_Original"() -> (w377:T1)
                  n185 = local read "MDF"() -> (w376:T1)
                  n186 = Not(x=w393) -> (.not. x?=w394:bool)
                  n187 = Not(x="Pause") -> (.not. x?=w381:bool)
                  n188 = Select(t=w377, s="Rerun MDF", f=w376) -> (s? t:f=w374:T1)
                  n189 = local read "RunAutoMode"() -> (w396:bool)
                  n190 = Or(x=w381, y="E-Stop") -> (x .or. y?=w379:bool)
                  n191 = Not(x=w379) -> (.not. x?=w378:bool)
                  n192 = local read "Where? Forebrain"() -> (w392:T2)
                  n193 = local read "What?Forebrain"() -> (w391:cluster{"T":dbl, "Range":dbl, "Bearing":dbl}[])
                  n194 = Boolean To (0,1)(Boolean=w378) -> (0, 1=w384:i16)
                  n195 = To Double Precision Float(number=w384) -> (double precision float=w383:dbl)
                  n196 = call "GotoWaypoint.vi"("SupressIn"=w383, "InhibitIn"=FALSE, "CurrentSteerAngle"=w385, "WhatAroundMe? Clean"=w391, "WhereAmI? Clean"=w392, "MDF In"=w374) -> ("MDF Out"=w388:T1, "ActCommand"=→"NeoActCom":dbl[], "Vel"=→"A Speed":dbl, "SteerAngle"=w386:dbl)  [unwired: 2 out]
                  "SteerAngle" <- w386
                  "MDF Out" <- w388
                  n197 = local write "MDF"(w388) -> ()
                  n198 = Wait (ms)(milliseconds to wait=u32 100) -> ()  [unwired: 1 out]
                  "Neo-C" <- w393
                }
                n199 = while {
                  shift-right: [w337] -> _
                  shift-left: _ -> [w332]
                  stop <- w331 stop-if-true
                  # "HowAmI?"
                  n200 = shared-variable "My Computer\\RobotBrainExLibrary.lvlib\\HowAmI? Clean"() -> (w333:cluster{"T":dbl, "Battery":dbl, "Temp":dbl})  [unwired: 1 in, 1 out]
                  "How?Midbrain" <- w333
                  n201 = call "HowForebrainPerception.vi"("How?MidbrainIn"=w333) -> ("TempWarning"=→"ATempLight":bool, "How?ForebrainOut"=→"How?Forebrain":cluster{"T":dbl, "Battery":dbl, "Temp":dbl}, "BatteryGauge"=→"AutoBattery":dbl)  [unwired: 1 in]
                  n202 = local read "RunAutoMode"() -> (w331:bool)
                  n203 = Not(x=w332) -> (.not. x?=w337:bool)
                  n204 = Wait (ms)(milliseconds to wait=u32 1000) -> ()  [unwired: 1 out]
                  "How?" <- w332
                }
                n205 = while {
                  shift-right: [w321] -> _
                  shift-left: _ -> [w322]
                  stop <- w324 stop-if-true
                  # "HypoThallumus"
                  n206 = Not(x=w322) -> (.not. x?=w321:bool)
                  n207 = local read "RunAutoMode"() -> (w324:bool)
                  n208 = call "Hypo-T.vi"() -> ("Act Out"=→"Hypo Out":cluster{"Motor1":i16, "Motor 2":i16})  [unwired: 3 in]
                  n209 = Wait (ms)(milliseconds to wait=u32 800) -> ()  [unwired: 1 out]
                  "Hypo" <- w322
                }
                n210 = while {
                  shift-right: [w329] -> _
                  shift-left: _ -> [w328]
                  stop <- w327 stop-if-true
                  # "ForebrainAct"
                  n211 = local read "NeoActCom"() -> (w326:dbl[])
                  n212 = local read "RunAutoMode"() -> (w327:bool)
                  n213 = Not(x=w328) -> (.not. x?=w329:bool)
                  n214 = call "ForebrainArbiter.vi"("WaypointInput"=w326) -> ("ForebrainActCom"=w325:dbl[])  [unwired: 14 in]
                  n215 = shared-variable "My Computer\\RobotBrainExLibrary.lvlib\\ActCommand"(w325) -> ()  [unwired: 1 in, 1 out]
                  n216 = Wait (ms)(milliseconds to wait=u32 100) -> ()  [unwired: 1 out]
                  "Act" <- w328
                }
              }
              frame #2 {
                w402 = T3."Startup&Shutdown" ("Tab")
                # "Set robot Vel to 0"
                # "Reset latched run\nswitch"
                # "Force control to\nShutdown Case"
                n217 = shared-variable "My Computer\\RobotBrainExLibrary.lvlib\\ForebrainCom"(T9 {"VelCom"=0.0, "BehCom"=enum."OpenFieldTransit"} ("ForebrainCom")) -> ()  [unwired: 1 in, 1 out]
                n218 = local write "RunAutoMode"(TRUE ("RunAutoMode")) -> ()
                n219 = Initialize Array(0.0 ("element"), 90 ("dimension size")) -> (w398:dbl[])
                n220 = shared-variable "My Computer\\RobotBrainExLibrary.lvlib\\ActCommand"(w398) -> ()  [unwired: 1 in, 1 out]
                n221 = local write "Tab"(w402) -> ()
              }
            }
          }
          frame "Documentation" {
            n222 = Wait (ms)(milliseconds to wait=u32 500) -> ()  [unwired: 1 out]
          }
          frame "DebugTHINK" {
            w412 = T3."Startup&Shutdown" ("Tab")
            # "Put code here in place of delay"
            # "Sends Tab Control\nback to Startup\ncase"
            n223 = Wait (ms)(milliseconds to wait=u32 2000) -> ()  [unwired: 1 out]
            n224 = local write "Tab"(w412) -> ()
          }
        }
        n225 = Not(x=w48) -> (.not. x?=w31:bool)
        "Robot Live" <- w31
      }
    }
    frame #2 {
      # "Realease LIDAR\nMemory"
      # "Reset Run \nSwitch"
      # "Shutdown Robot"
      n226 = call "Pixel_LIDAR_Close.vi"("error in (no error) 2"=w414, "Image"=w415) -> ()  [unwired: 1 in]
      n227 = local write "RunRobot"(TRUE ("RunRobot")) -> ()
    }
  }
